vi "WinCI Not A Source Control Reference.vi"(8 "error in (no error)":errorcluster, 10 "source control reference in":T1) -> (0 "error out":errorcluster, 2 "not a source control reference?":bool)   [LabVIEW 2017, in "NI_SCC_WinCI.lvlib"]
doc: "Returns TRUE if <B>semaphore</B> is not a valid semaphore refnum."
uses:
  <vilib>/SourceControl/Providers/WinCI/NI_SCC_WinCI.lvlib
  <vilib>/SourceControl/sccapi/SCCAPI Refnum.ctl
  <vilib>/SourceControl/sccapi/NI_SCC.lvlib
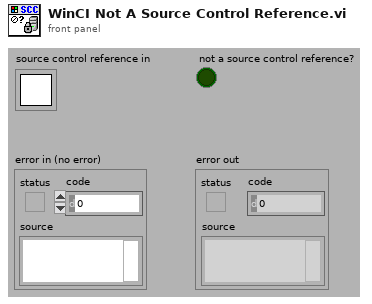
[diagram p1: front panel]
types:
  T1 = typedef "NI_SCC.lvlib/SCCAPI Refnum.ctl" = refnum<k1>
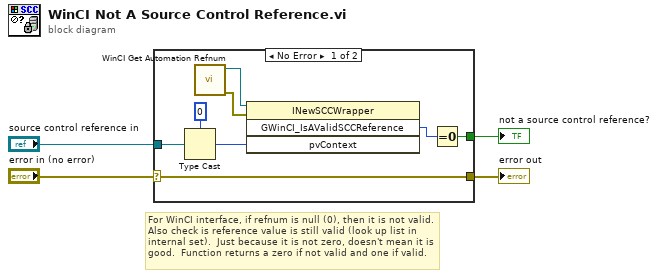
[diagram p0: block diagram]
diagram:
  # "For WinCI interface, if refnum is null (0), then it is not valid.  Also check is reference value is still valid (look up list in internal set).  Just because it is not zero, doesn't mean it is good.  Function returns a zero if not valid and one if valid."
  n1 = case shown="No Error" "error in (no error)" {
    selector: "error in (no error)" -> [w10 w13]
    tunnel: [w10 w13] -> w4
    tunnel: [w9 _] -> w3
    tunnel: "source control reference in" -> [w12 _]
    frame No Error {
      n2 = Type Cast(type=u32 0, x=w12) -> (*(type *) &x=w7:u32)
      n3 = call <vilib>:"WinCI Get Automation Refnum.vi"() -> ("error out"=w5:errorcluster, "automation refnum"=w6:refnum<k7>)  [unwired: 10 out]
      n4 = invoke class="INewSCCWrapper" method="GWinCI_IsAValidSCCReference"(reference=w6, error in=w5, "pvContext"=w7) -> ("GWinCI_IsAValidSCCReference"=w8:i32)  [unwired: 1 in, 3 out]
      n5 = Equal To 0?(x=w8) -> (x = 0?=w9:bool)
    }
    frame Error {
      # "Return false if there was an error.  Since we never test refnum, we can't say if it's bad."
    }
  }
  "not a source control reference?" <- w3
  "error out" <- w4
